vi "test Listen Only.vi"(11 "Test Case In":refnum<class "Test PCANBasic.lvclass">) -> (0 "error out":errorcluster, 3 "Test Case Out":refnum<class "Test PCANBasic.lvclass">)   [LabVIEW 2020, in "Test PCANBasic.lvclass"]
uses:
  Test PCANBasic.lvclass
  Test PCANBasic.lvclass/Test PCANBasic.ctl
  C:/Program Files/National Instruments/LabVIEW 2026/vi.lib/Astemes/LUnit/Test Case.lvclass
  C:/Program Files/National Instruments/LabVIEW 2026/vi.lib/Astemes/LUnit/LUnit Runnable.lvclass
  D:/git/PCAN-Basic-LabVIEW/tests/Tests PCANBasic/Test PCANBasic.lvclass
  source/PCANBasic.lvlib
  <vilib>/Astemes/LUnit/Test Case.lvclass
  Global PCAN Channel.vi
  Global PCAN Baudrate.vi
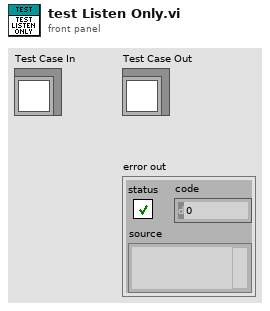
[diagram p1: front panel]
types:
  T1 = typedef "PCANBasic.lvlib/TPCANHandle.ctl" = u16
  T2 = typedef "PCANBasic.lvlib/PCAN Baud.ctl" = u16
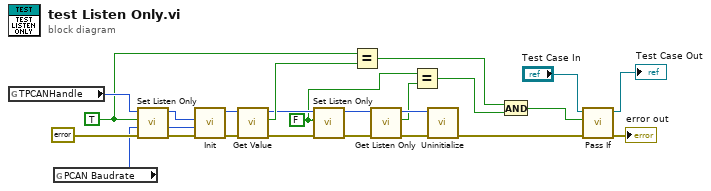
[diagram p0: block diagram]
diagram:
  w3 = FALSE ("Enable")
  w4 = TRUE ("Enable")
  n1 = global read "Global PCAN Channel.vi" "TPCANHandle"() -> (w13:T1)
  n2 = global read "Global PCAN Baudrate.vi" "PCAN Baudrate"() -> (w17:T2)
  n3 = call "Set Listen Only.vi"("error in"=errorcluster {"status"=FALSE, "code"=0, "source"=""}, "Enable"=w4, "TPCANHandle in"=w13) -> ("error out"=w14:errorcluster, "TPCANHandle out"=w12:T1)  [unwired: 6 in, 1 out]
  n4 = call "Init.vi"("error in"=w14, "Baudrate"=w17, "Channel"=w12) -> ("error out"=w19:errorcluster, "TPCANHandle out"=w18:T1)  [unwired: 6 in, 1 out]
  n5 = call-poly "Get Value.vi"("error in"=w19, "TPCANHandle in"=w18) -> ("error out"=w21:errorcluster, "Enabled"=w15:bool, "TPCANHandle out"=w10:T1)  [unwired: 6 in, 1 out]
  n6 = call "Set Listen Only.vi"("error in"=w21, "Enable"=w3, "TPCANHandle in"=w10) -> ("error out"=w11:errorcluster, "TPCANHandle out"=w7:T1)  [unwired: 6 in, 1 out]
  n7 = Equal?(x=w4, y=w15) -> (x = y?=w1:bool)
  n8 = call "Get Listen Only.vi"("error in"=w11, "TPCANHandle in"=w7) -> ("error out"=w8:errorcluster, "Enabled"=w5:bool, "TPCANHandle out"=w6:T1)  [unwired: 6 in, 1 out]
  n9 = Equal?(x=w3, y=w5) -> (x = y?=w9:bool)
  n10 = call "Uninitialize.vi"("error in"=w8, "TPCANHandle in"=w6) -> ("error out"=w16:errorcluster)  [unwired: 8 in, 1 out]
  n11 = And(x=w1, y=w9) -> (x .and. y?=w2:bool)
  n12 = call <vilib>:"Pass If.vi"("error in (no error)"=w16, "Pass?"=w2, "LUnit Test Case In"="Test Case In") -> ("error out"=→"error out":errorcluster, "LUnit Test Case Out"=→"Test Case Out":refnum<class "Test PCANBasic.lvclass">)  [unwired: 7 in]
